vi "TimerG.vi"() -> ()   [LabVIEW 2020, in "Timer.lvlib"]
uses:
  Timer.lvlib
panel:
  in  "Timer":map{string, dbl}(c390)
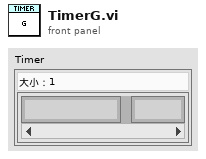
[diagram p1: front panel]
diagram:
